vi "Metronome.vi"() -> ()   [LabVIEW 2015]
panel:
  in  "stop":bool
  in  "Beats Per Minute":dbl
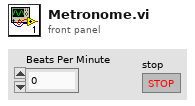
[diagram p1: front panel]
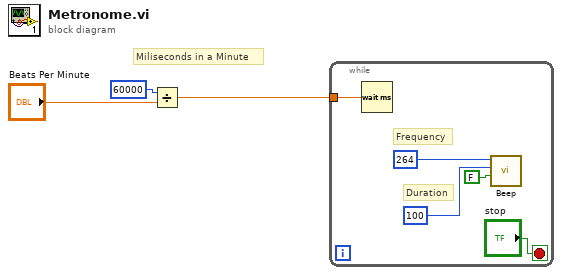
[diagram p0: block diagram]
diagram:
  # "Miliseconds in a Minute"
  n1 = Divide(x=60000, y="Beats Per Minute") -> (x/y=w1:dbl)
  n2 = while {
    tunnel: w1 -> [w4]
    stop <- "stop" stop-if-true
    # "Duration"
    # "Frequency"
    n3 = Wait (ms)(milliseconds to wait=w4) -> ()  [unwired: 1 out]
    n4 = call <vilib>:"Beep.vi"("use system alert? (T)"=FALSE, "duration (msec)"=u32 100, "frequency (Hz)"=u32 264) -> ()  [unwired: 9 in]
  }
